vi "TMCL.vi"(0 "Address":i32, 1 "Instruction":i32, 2 "Type":i32, 3 "Motor":i32, 4 "Value":i32) -> (5 "Hexadecimal value":string, 6 "CRC (Optional)":i32)   [LabVIEW 2016]
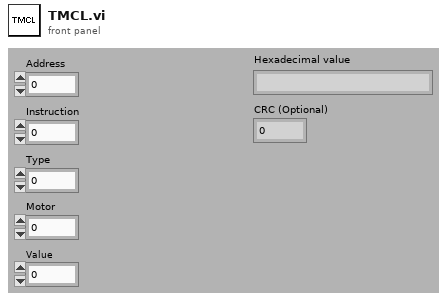
[diagram p1: front panel]
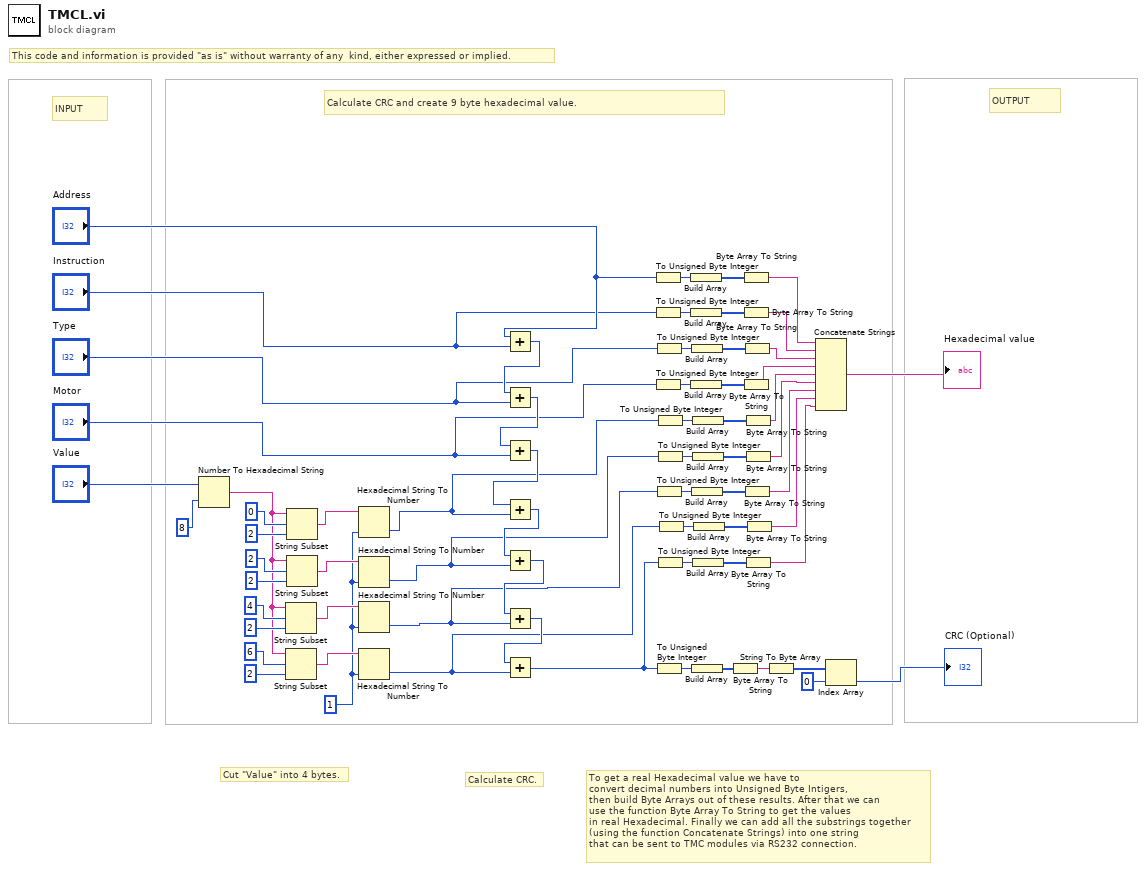
[diagram p0: block diagram]
diagram:
  w8 = 1
  # "This code and information is provided \"as is\" without warranty of any  kind, either expressed or implied."
  # "Calculate CRC."
  # "Cut \"Value\" into 4 bytes."
  # "Calculate CRC and create 9 byte hexadecimal value."
  # "OUTPUT"
  # "INPUT"
  # "To get a real Hexadecimal value we have to\nconvert decimal numbers into Unsigned Byte Intigers,\nthen build Byte Arrays out of these results. After that we can\nuse the function Byte Array To String to get the values \nin real Hexadecimal. Finally we can add all the substrings together\n(using the function Concatenate Strings) into one string\nthat can be sent to TMC modules via RS232 connection."
  n1 = Number To Hexadecimal String ("Numb To Hex")(1:8, 2:"Value") -> (0:w18:string)
  n2 = String Subset(string=w18, offset (0)=4, length (rest)=2) -> (substring=w27:string)
  n3 = String Subset(string=w18, offset (0)=6, length (rest)=2) -> (substring=w26:string)
  n4 = String Subset(string=w18, offset (0)=0, length (rest)=2) -> (substring=w29:string)
  n5 = String Subset(string=w18, offset (0)=2, length (rest)=2) -> (substring=w28:string)
  n6 = Hexadecimal String To Number(string=w29, default (0uL)=w8) -> (number=w9:i32)  [unwired: 1 in, 1 out]
  n7 = Hexadecimal String To Number(string=w28, default (0uL)=w8) -> (number=w10:i32)  [unwired: 1 in, 1 out]
  n8 = Hexadecimal String To Number(string=w27, default (0uL)=w8) -> (number=w11:i32)  [unwired: 1 in, 1 out]
  n9 = Hexadecimal String To Number(string=w26, default (0uL)=w8) -> (number=w12:i32)  [unwired: 1 in, 1 out]
  n10 = Add(x="Address", y="Instruction") -> (x+y=w25:i32)
  n11 = Add(x=w25, y="Type") -> (x+y=w24:i32)
  n12 = Add(x=w24, y="Motor") -> (x+y=w23:i32)
  n13 = Add(x=w23, y=w9) -> (x+y=w22:i32)
  n14 = Add(x=w22, y=w10) -> (x+y=w21:i32)
  n15 = Add(x=w21, y=w11) -> (x+y=w20:i32)
  n16 = Add(x=w20, y=w12) -> (x+y=w3:i32)
  n17 = To Unsigned Byte Integer(number="Address") -> (unsigned 8bit integer=w64:u8)
  n18 = To Unsigned Byte Integer(number="Instruction") -> (unsigned 8bit integer=w61:u8)
  n19 = To Unsigned Byte Integer(number="Motor") -> (unsigned 8bit integer=w45:u8)
  n20 = To Unsigned Byte Integer(number="Type") -> (unsigned 8bit integer=w59:u8)
  n21 = To Unsigned Byte Integer(number=w11) -> (unsigned 8bit integer=w51:u8)
  n22 = To Unsigned Byte Integer(number=w3) -> (unsigned 8bit integer=w7:u8)
  n23 = To Unsigned Byte Integer(number=w9) -> (unsigned 8bit integer=w57:u8)
  n24 = To Unsigned Byte Integer(number=w10) -> (unsigned 8bit integer=w53:u8)
  n25 = To Unsigned Byte Integer(number=w3) -> (unsigned 8bit integer=w42:u8)
  n26 = To Unsigned Byte Integer(number=w12) -> (unsigned 8bit integer=w49:u8)
  n27 = Build Array(w64) -> (w65:u8[])
  n28 = Build Array(w61) -> (w62:u8[])
  n29 = Build Array(w45) -> (w44:u8[])
  n30 = Build Array(w59) -> (w58:u8[])
  n31 = Build Array(w51) -> (w50:u8[])
  n32 = Build Array(w7) -> (w6:u8[])
  n33 = Build Array(w57) -> (w56:u8[])
  n34 = Build Array(w53) -> (w52:u8[])
  n35 = Build Array(w42) -> (w39:u8[])
  n36 = Build Array(w49) -> (w48:u8[])
  n37 = Byte Array To String(unsigned byte array=w6) -> (string=w2:string)
  n38 = Byte Array To String(unsigned byte array=w65) -> (string=w63:string)
  n39 = Byte Array To String(unsigned byte array=w62) -> (string=w60:string)
  n40 = Byte Array To String(unsigned byte array=w44) -> (string=w43:string)
  n41 = Byte Array To String(unsigned byte array=w58) -> (string=w55:string)
  n42 = Byte Array To String(unsigned byte array=w50) -> (string=w46:string)
  n43 = Byte Array To String(unsigned byte array=w56) -> (string=w54:string)
  n44 = Byte Array To String(unsigned byte array=w52) -> (string=w47:string)
  n45 = Byte Array To String(unsigned byte array=w39) -> (string=w41:string)
  n46 = Byte Array To String(unsigned byte array=w48) -> (string=w40:string)
  n47 = String To Byte Array(string=w2) -> (unsigned byte array=w4:u8[])
  n48 = Concatenate Strings(w63, w60, w55, w43, w54, w47, w46, w40, w41) -> (→"Hexadecimal value":string)
  n49 = Index Array(array=w4, index=0 ("Index")) -> (element=→"CRC (Optional)":u8)
